vi "Control Panel.vi"() -> ()   [LabVIEW 2017, in "HP4192A IA.lvclass"]
uses:
  HP4192A IA.lvclass
  Global/GPIB Numbers.vi
  Scan.vi
panel:
  in  "?":bool
  out "Unit C":enum16{"kHz", "V", "mA", "Reference Data"}(ring)
  in  "Function B":u16(ring) items=["DEG, Q", "RAD, D", "R/G"]
  in  "Function A":u16(ring) items=["Z/Y", "R/G", "L", "C"]
  out "Reading":bool
  in  "Averaging":i16(slide) scale=0.0..1.0
  out "Overflow":bool
  out "Overflow":bool
  in  "OSC Level":dbl
  in  "?":bool
  in  "Set Frequency":dbl=1000.0 min=0.0 max=13000000.0 format="%#_6e"
  in  "DC Bias?":bool
  in  "Bias":dbl
  in  "Trigger":u16(ring) items=["Internal", "External", "Hold/Manual"]
  in  "Circuit Mode":enum32{"Auto", "Series", "Parallel"}(ring)
  out "Display C":dbl
  out "Display B":dbl
  out "Display A":dbl
  # "V"
  # "V"
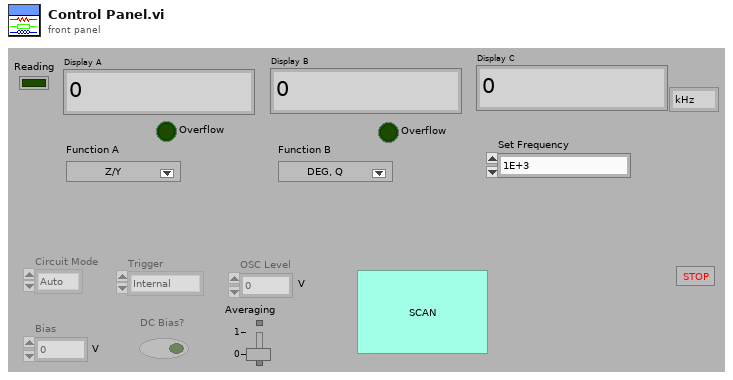
[diagram p1: front panel]
types:
  T1 = typedef "GPIB Type Def.ctl" = cluster{"Name":string, "bus":dbl, "GPIB":dbl, "GPIB as string":string, "byte":i32, "VISA Resource Name":refnum<visa-resource-name>}
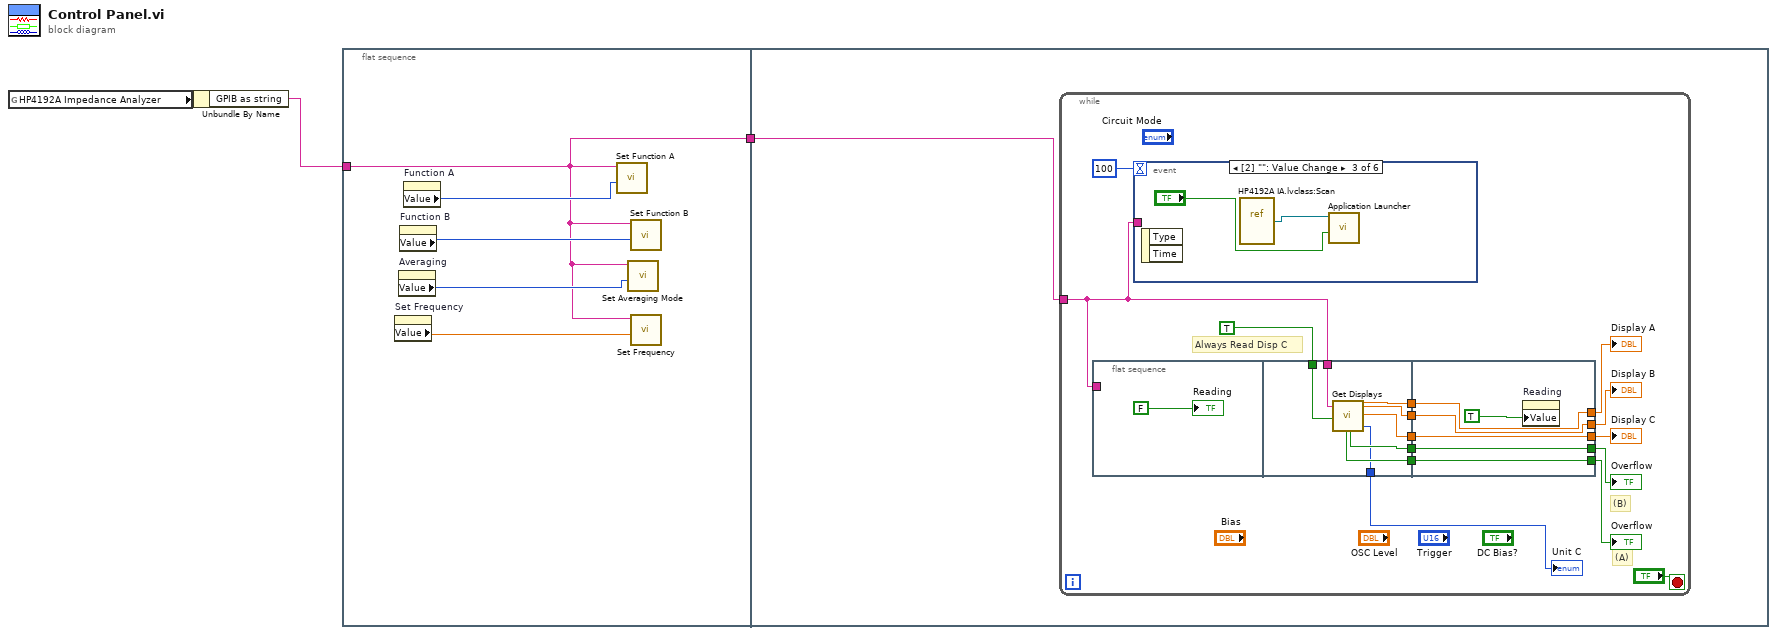
[diagram p0: block diagram]
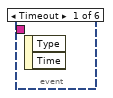
[diagram p2: hidden frame]
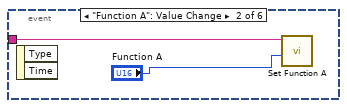
[diagram p3: hidden frame]
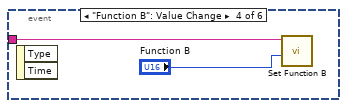
[diagram p4: hidden frame]
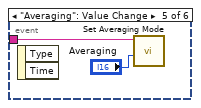
[diagram p5: hidden frame]
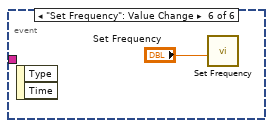
[diagram p6: hidden frame]
diagram:
  n1 = global read "GPIB Numbers.vi" "HP4192A Impedance Analyzer"() -> (w3:T1)
  n2 = Unbundle By Name(w3) -> ("GPIB as string"=w2:string)
  n3 = flat-sequence {
    tunnel: w2 -> [w5]
    tunnel: [w5] -> w1
    tunnel: w1 -> [w9]
    frame #0 {
      n4 = property on="Set Frequency" class="DigNum (strict)"() -> ("Value"=w4:dbl[unit])  [unwired: 2 in, 2 out]
      n5 = property on="Averaging" class="Slide (strict)"() -> ("Value"=w6:i16)  [unwired: 2 in, 2 out]
      n6 = property on="Function B" class="Ring (strict)"() -> ("Value"=w7:u16)  [unwired: 2 in, 2 out]
      n7 = property on="Function A" class="Ring (strict)"() -> ("Value"=w8:u16)  [unwired: 2 in, 2 out]
      n8 = call "Set Function A.vi"("function A (z/y:0)"=w8, "GPIB addess"=w5) -> ()  [unwired: 10 in]
      n9 = call "Set Averaging Mode.vi"("Averaging"=w6, "GPIB addess"=w5) -> ()  [unwired: 10 in]
      n10 = call "Set Function B.vi"("function B (deg q:0)"=w7, "GPIB addess"=w5) -> ()  [unwired: 10 in]
      n11 = call "Set Frequency.vi"("test signal\nfreq (Hz)"=w4, "GPIB addess"=w5) -> ()  [unwired: 10 in]
    }
    frame #1 {
      n12 = while {
        tunnel: w9 -> [w17]
        stop <- "?" stop-if-true
        # "Always Read Disp C"
        # "(A)"
        # "(B)"
        n13 = flat-sequence {
          tunnel: w17 -> [_]
          tunnel: w17 -> [w42]
          tunnel: TRUE -> [w36]
          tunnel: [w41] -> w16
          tunnel: [w40] -> w15
          tunnel: [w39] -> w14
          tunnel: [w38] -> w13
          tunnel: [w37] -> w12
          tunnel: [w35] -> w10
          tunnel: [w44] -> w19
          tunnel: [w45] -> w20
          tunnel: [w46] -> w21
          tunnel: [w47] -> w22
          tunnel: [w48] -> w23
          tunnel: w16 -> [w48]
          tunnel: w15 -> [w47]
          tunnel: w14 -> [w46]
          tunnel: w13 -> [w45]
          tunnel: w12 -> [w44]
          frame #0 {
            "Reading" <- FALSE
          }
          frame #1 {
            n14 = call "Get Displays.vi"("GPIB addess"=w42, "Read C?"=w36) -> ("A Overflow"=w38:bool, "B Overflow"=w37:bool, "display A"=w41:dbl, "display B"=w40:dbl, "display C"=w39:dbl, "Unit C"=w35:enum16{"kHz", "V", "mA", "Reference Data"})  [unwired: 17 in, 3 out]
          }
          frame #2 {
            n15 = property on="Reading" class="Bool (strict)"("Value"=TRUE) -> ()  [unwired: 2 in, 2 out]
          }
        }
        n16 = event shown="[2] \"\": Value Change" {
          selector: _ -> [_ _ _ _ _ _]
          dyn-events: _ -> [_ _ _ _ _ _]
          timeout: 100 -> [_ _ _ _ _ _]
          tunnel: w17 -> [_ w26 _ w30 w31 _]
          event Timeout {
            n17 = event-data() -> ()  [unwired: 1 in, 2 out]
          }
          event "Function A": Value Change {
            n18 = event-data() -> ()  [unwired: 1 in, 2 out]
            n19 = call "Set Function A.vi"("function A (z/y:0)"="Function A", "GPIB addess"=w26) -> ()  [unwired: 10 in]
          }
          event Value Change {
            n20 = event-data() -> ()  [unwired: 1 in, 2 out]
            n21 = vi-ref "HP4192A IA.lvclass:Scan.vi"() -> (w28:refnum<vi>)
            n22 = call "Application Launcher.vi"("Toggle?"="?", "VI reference"=w28) -> ()  [unwired: 1 in, 9 out]
          }
          event "Function B": Value Change {
            n23 = event-data() -> ()  [unwired: 1 in, 2 out]
            n24 = call "Set Function B.vi"("function B (deg q:0)"="Function B", "GPIB addess"=w30) -> ()  [unwired: 10 in]
          }
          event "Averaging": Value Change {
            n25 = event-data() -> ()  [unwired: 1 in, 2 out]
            n26 = call "Set Averaging Mode.vi"("Averaging"="Averaging", "GPIB addess"=w31) -> ()  [unwired: 10 in]
          }
          event "Set Frequency": Value Change {
            n27 = event-data() -> ()  [unwired: 1 in, 2 out]
            n28 = call "Set Frequency.vi"("test signal\nfreq (Hz)"="Set Frequency") -> ()  [unwired: 11 in]
          }
        }
        "Display A" <- w23
        "Display B" <- w22
        "Display C" <- w21
        "Overflow" <- w19
        "Overflow" <- w20
        "Unit C" <- w10
      }
    }
  }
